vi "my_std_dev2.vi"(7 "y":dbl, 11 "x":dbl) -> (5 "sqrt(x)":dbl)   [LabVIEW 2021]
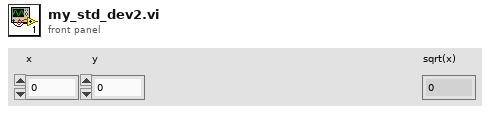
[diagram p1: front panel]
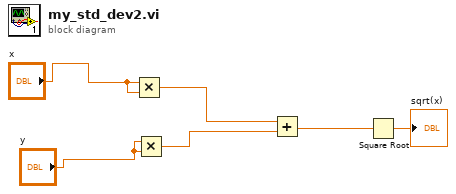
[diagram p0: block diagram]
diagram:
  n1 = Multiply(x="x", y="x") -> (x*y=w4:dbl)
  n2 = Multiply(x="y", y="y") -> (x*y=w5:dbl)
  n3 = Add(x=w4, y=w5) -> (x+y=w6:dbl)
  n4 = Square Root(x=w6) -> (sqrt(x)=→"sqrt(x)":dbl)
